vi "P2Judge Queue Management.vi"(6 "Mode":T2, 8 "error in":errorcluster, 9 "Variant Data":variant, 10 "Command":string, 11 "Queue Index":T1) -> (0 "error out":errorcluster, 1 "Status":bool[](array[boolean]), 3 "Queue":refnum<queue>)   [LabVIEW 2016]
uses:
  controls/P2Judge QueueCtl.ctl
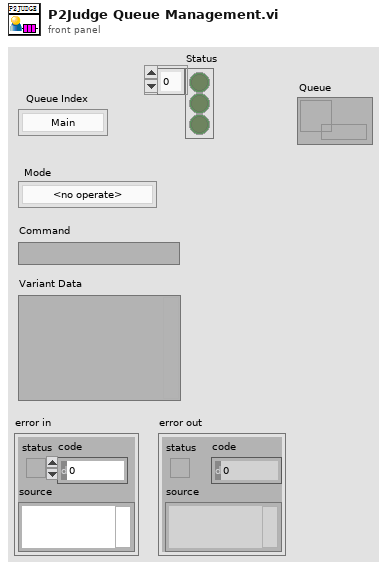
[diagram p1: front panel]
types:
  T1 = typedef "P2Judge QueueCtl.ctl" = enum16{"Main", "Device", "Picture"}
  T2 = typedef "QueueModeCtl.ctl" = enum16{"<no operate>", "Send", "Send(head)", "Flush", "Destory", "Send>All", "Send>All(head)", "Flush All", "Destory All"}
  T3 = typedef "QueueDataCtl.ctl" = cluster{"Command":string, "Variant Data":variant}
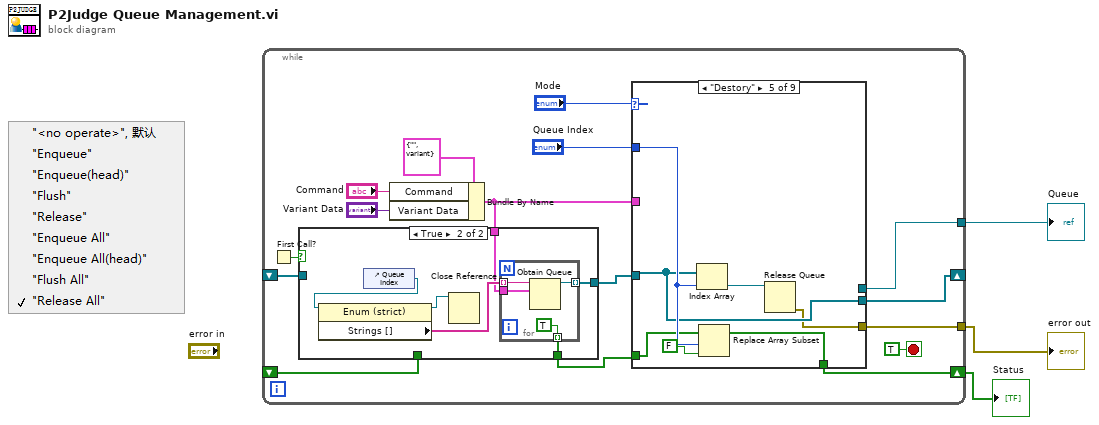
[diagram p0: block diagram]
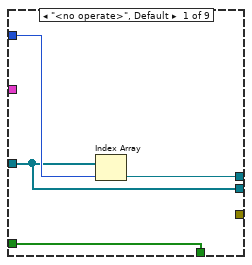
[diagram p2: hidden frame]
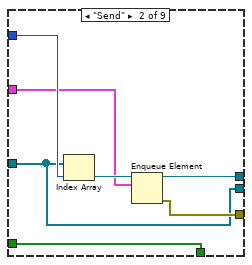
[diagram p3: hidden frame]
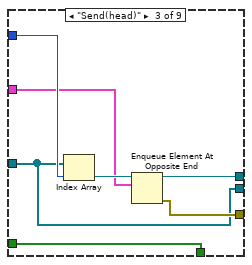
[diagram p4: hidden frame]
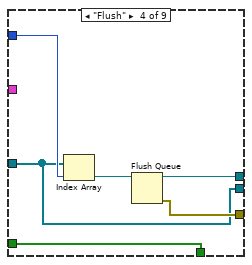
[diagram p5: hidden frame]
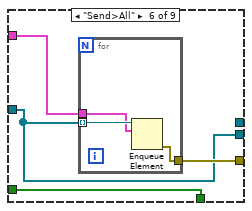
[diagram p6: hidden frame]
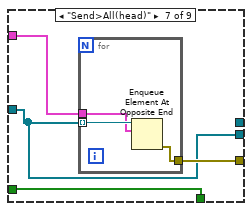
[diagram p7: hidden frame]
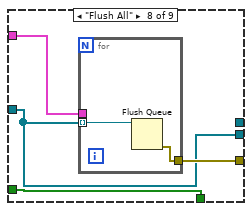
[diagram p8: hidden frame]
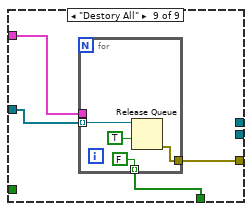
[diagram p9: hidden frame]
diagram:
  n1 = while {
    shift-right: [w7] -> _
    shift-left: _ -> [w19]
    tunnel: [w9] -> w3
    tunnel: [w8] -> w2
    shift-right: [w5] -> w1
    shift-left: _ -> [w4]
    stop <- TRUE stop-if-true
    n2 = First Call?() -> (First Call?: T/F=w14:bool)
    n3 = Bundle By Name(cluster=T3 {"Command"="", "Variant Data"=variant} ("main window queue data"), "Command"="Command", "Variant Data"="Variant Data") -> (w12:T3)
    n4 = case shown="True" w14 {
      tunnel: w19 -> [w80 _]
      tunnel: w12 -> [_ w83]
      tunnel: [w80 w82] -> w11
      tunnel: [w79 w81] -> w6
      tunnel: w4 -> [w79 _]
      frame False {
      }
      frame True {
        n5 = control-ref of="Queue Index"() -> (w86:refnum<vi>)
        n6 = property class="Enum (strict)"(reference=w86) -> (reference out=w85:refnum<vi>, "Strings []"=w84:string[])  [unwired: 1 in, 1 out]
        n7 = Close Reference(reference=w85) -> ()  [unwired: 1 in, 1 out]
        n8 = for {
          tunnel: w84 -> [w89] mode=indexing
          tunnel: w83 -> [w90]
          tunnel: [w88] -> w82 mode=indexing
          tunnel: [TRUE] -> w81 mode=indexing
          n9 = Obtain Queue(name (unnamed)=w89, element data type=w90) -> (queue out=w88:refnum<queue>)  [unwired: 3 in, 2 out]
        }
      }
    }
    n10 = case shown="\"Destory\"" "Mode" {
      tunnel: w12 -> [_ w28 w35 _ _ w53 w60 w67 w72]
      tunnel: w11 -> [w21 w25 w32 w39 w47 w52 w59 w66 w73]
      tunnel: "Queue Index" -> [w23 w30 w37 w43 w49 _ _ _ _]
      tunnel: [_ w27 w34 w41 w46 w54 w61 w68 w74] -> w9
      tunnel: [w22 w26 w33 w40 _ _ _ _ _] -> w8
      tunnel: [w21 w25 w32 w39 w47 w52 w59 w66 _] -> w7
      tunnel: w6 -> [w20 w24 w31 w38 w45 w51 w58 w65 _]
      tunnel: [w20 w24 w31 w38 w44 w51 w58 w65 w71] -> w5
      frame "<no operate>", Default {
        n11 = Index Array(array=w21, index=w23) -> (element=w22:refnum<queue>)
      }
      frame "Send" {
        n12 = Index Array(array=w25, index=w30) -> (element=w29:refnum<queue>)
        n13 = Enqueue Element(queue=w29, element=w28) -> (queue out=w26:refnum<queue>, error out=w27:errorcluster)  [unwired: 2 in, 1 out]
      }
      frame "Send(head)" {
        n14 = Index Array(array=w32, index=w37) -> (element=w36:refnum<queue>)
        n15 = Enqueue Element At Opposite End(queue=w36, element=w35) -> (queue out=w33:refnum<queue>, error out=w34:errorcluster)  [unwired: 2 in, 1 out]
      }
      frame "Flush" {
        n16 = Index Array(array=w39, index=w43) -> (element=w42:refnum<queue>)
        n17 = Flush Queue(queue=w42) -> (queue out=w40:refnum<queue>, error out=w41:errorcluster)  [unwired: 1 in, 1 out]
      }
      frame "Destory" {
        n18 = Index Array(array=w47, index=w49) -> (element=w48:refnum<queue>)
        n19 = Replace Array Subset(array=w45, new element=FALSE, index=w49) -> (w44:bool[])
        n20 = Release Queue(queue=w48) -> (error out=w46:errorcluster)  [unwired: 2 in, 2 out]
      }
      frame "Send>All" {
        n21 = for {
          tunnel: [w57] -> w54
          tunnel: w52 -> [w56] mode=indexing
          tunnel: w53 -> [w55]
          n22 = Enqueue Element(queue=w56, element=w55) -> (error out=w57:errorcluster)  [unwired: 2 in, 2 out]
        }
      }
      frame "Send>All(head)" {
        n23 = for {
          tunnel: [w64] -> w61
          tunnel: w59 -> [w63] mode=indexing
          tunnel: w60 -> [w62]
          n24 = Enqueue Element At Opposite End(queue=w63, element=w62) -> (error out=w64:errorcluster)  [unwired: 2 in, 2 out]
        }
      }
      frame "Flush All" {
        n25 = for {
          tunnel: [w70] -> w68
          tunnel: w66 -> [w69] mode=indexing
          tunnel: w67 -> [_]
          n26 = Flush Queue(queue=w69) -> (error out=w70:errorcluster)  [unwired: 1 in, 2 out]
        }
      }
      frame "Destory All" {
        n27 = for {
          tunnel: [w78] -> w74
          tunnel: w73 -> [w77] mode=indexing
          tunnel: w72 -> [_]
          tunnel: [FALSE] -> w71 mode=indexing
          n28 = Release Queue(queue=w77, force destroy? (F)=TRUE ("强制销毁？(F)")) -> (error out=w78:errorcluster)  [unwired: 1 in, 2 out]
        }
      }
    }
  }
  "error out" <- w3
  "Queue" <- w2
  "Status" <- w1
